vi "FPGA_I2C_AD7747_Write_Read.vi"(5 "SPI Command":string="0000", 6 "SelectDut":bool[][](array[boolean])=[[TRUE, TRUE, TRUE, TRUE, TRUE, TRUE, TRUE, TRUE, TRUE, TRUE, TRUE, TRUE, TRUE, TRUE, TRUE, TRUE, FALSE, FALSE, FALSE, FALSE, FALSE, FALSE, FALSE, FALSE, FALSE, FALSE, FALSE, FALSE, FALSE, FALSE, FALSE, FALSE], [TRUE, TRUE, TRUE, TRUE, TRUE, TRUE, TRUE, TRUE, TRUE, TRUE, TRUE, TRUE, TRUE, TRUE, TRUE, TRUE, FALSE, FALSE, FALSE, FALSE, FALSE, FALSE, FALSE, FALSE, FALSE, FALSE, FALSE, FALSE, FALSE, FALSE, FALSE, FALSE], [FALSE, FALSE, FALSE, FALSE, FALSE, FALSE, FALSE, FALSE, FALSE, FALSE, FALSE, FALSE, FALSE, FALSE, FALSE, FALSE, TRUE, FALSE, FALSE, FALSE, FALSE, FALSE, TRUE, FALSE, FALSE, FALSE, FALSE, FALSE, FALSE, FALSE, FALSE, TRUE], [FALSE, FALSE, FALSE, FALSE, FALSE, FALSE, FALSE, FALSE, FALSE, FALSE, FALSE, FALSE, FALSE, FALSE, FALSE, FALSE, TRUE, FALSE, FALSE, FALSE, FALSE, FALSE, TRUE, FALSE, FALSE, FALSE, FALSE, FALSE, FALSE, FALSE, FALSE, TRUE]], 7 "Stop":bool, 8 "error in":errorcluster, 9 "OFFSet Cal":bool, 10 "CapDac":bool, 11 "READ":bool) -> (0 "error out":errorcluster, 2 "Cap_Data":string[][](table)=[["0x02", "3.76992", "0x02", "3.77728"], ["0x02", "3.78382", "0x00", "-8.19200"], ["0x02", "3.94961", "0x02", "3.76741"], ["0x02", "4.54733", "0x02", "4.63408"], ["0x02", "3.84893", "0x02", "3.82712"], ["0x02", "3.80094", "0x02", "3.80246"], ["0x02", "3.79069", "0x02", "3.74972"], ["0x02", "3.80074", "0x02", "3.79936"], ["0x02", "4.04241", "0x02", "3.22665"], ["0x02", "3.79415", "0x02", "3.76417"], ["0x02", "3.79553", "0x02", "3.77940"], ["0x02", "1.03695", "0x02", "1.03735"], ["0x02", "3.80021", "0x02", "3.77078"], ["0x02", "4.65608", "0x02", "4.70829"], ["0x02", "3.74688", "0x02", "3.75749"], ["0x02", "3.81169", "0x02", "3.79781"]])   [LabVIEW 2012]
panel:
  out "Activity Log":string
  in  "Monitor":bool=TRUE
  in  "Write SPI":bool
  out "Simulate FPGA":bool
  out "Online":bool
  in  "SPI Clock Rate (Hz)":dbl=1000000.0 caption="Clock Rate" format="%.1p Hz"
  in  "I2C Slave Address":u8=144 caption="Slave Address" format="0x%02x"
  in  "I2C Clock Rate (Hz)":dbl=100000.0 caption="Clock Rate" format="%.0p Hz"
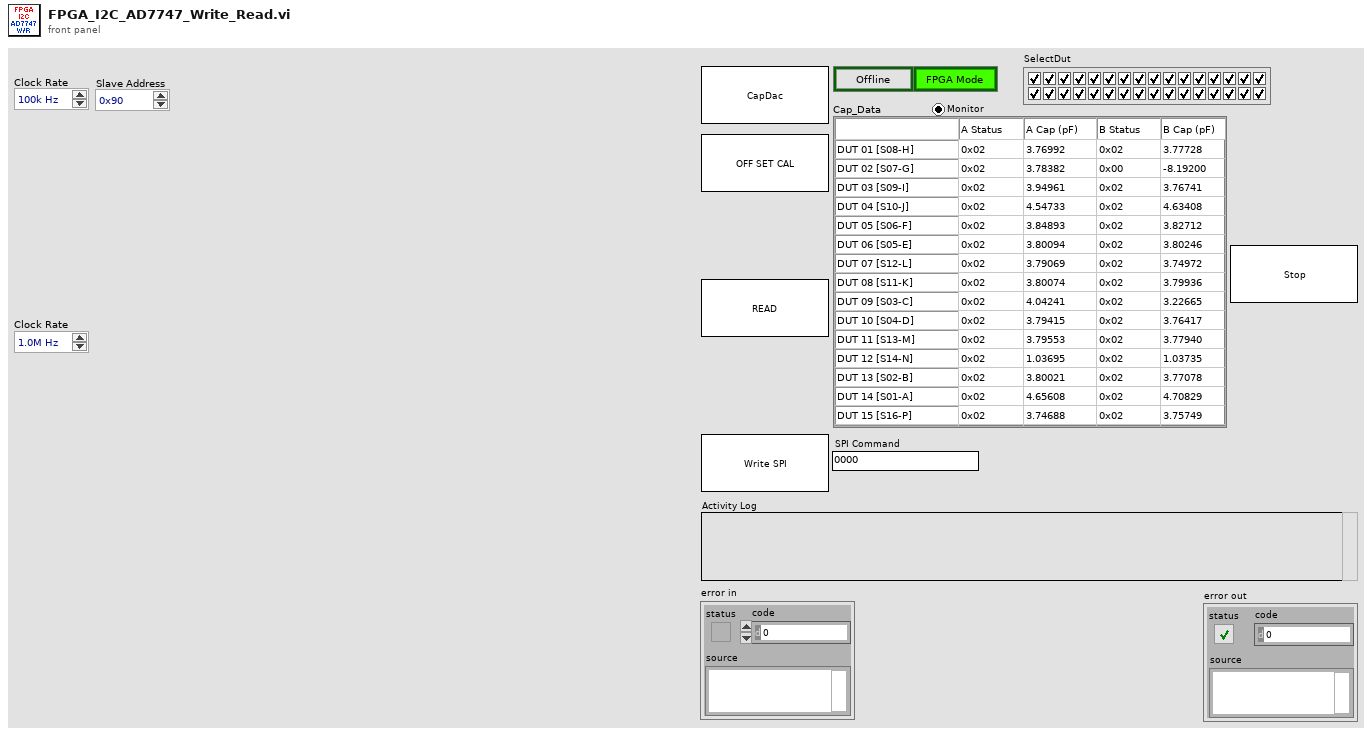
[diagram p1: front panel]
types:
  T1 = typedef "WSVCAP SHL Core System Cluster.ctl" = cluster{"Settings":T2, "FPGA Resource":tag, "Online":bool, "I2C Wait Ticks":u32, "SPI Wait Ticks":u32, "RFFE Wait Ticks":u32}
  T2 = typedef "WSVCAP SHL I2C Settings Cluster.ctl" = cluster{"FPGA Resource Name":string, "I2C Slave Address":u8, "I2C Clock Rate (Hz)":dbl, "SPI Clock Rate (Hz)":dbl, "RFFE Slave Address":u8, "RFFE Clock Rate (Hz)":dbl, "Simulate FPGA":bool}
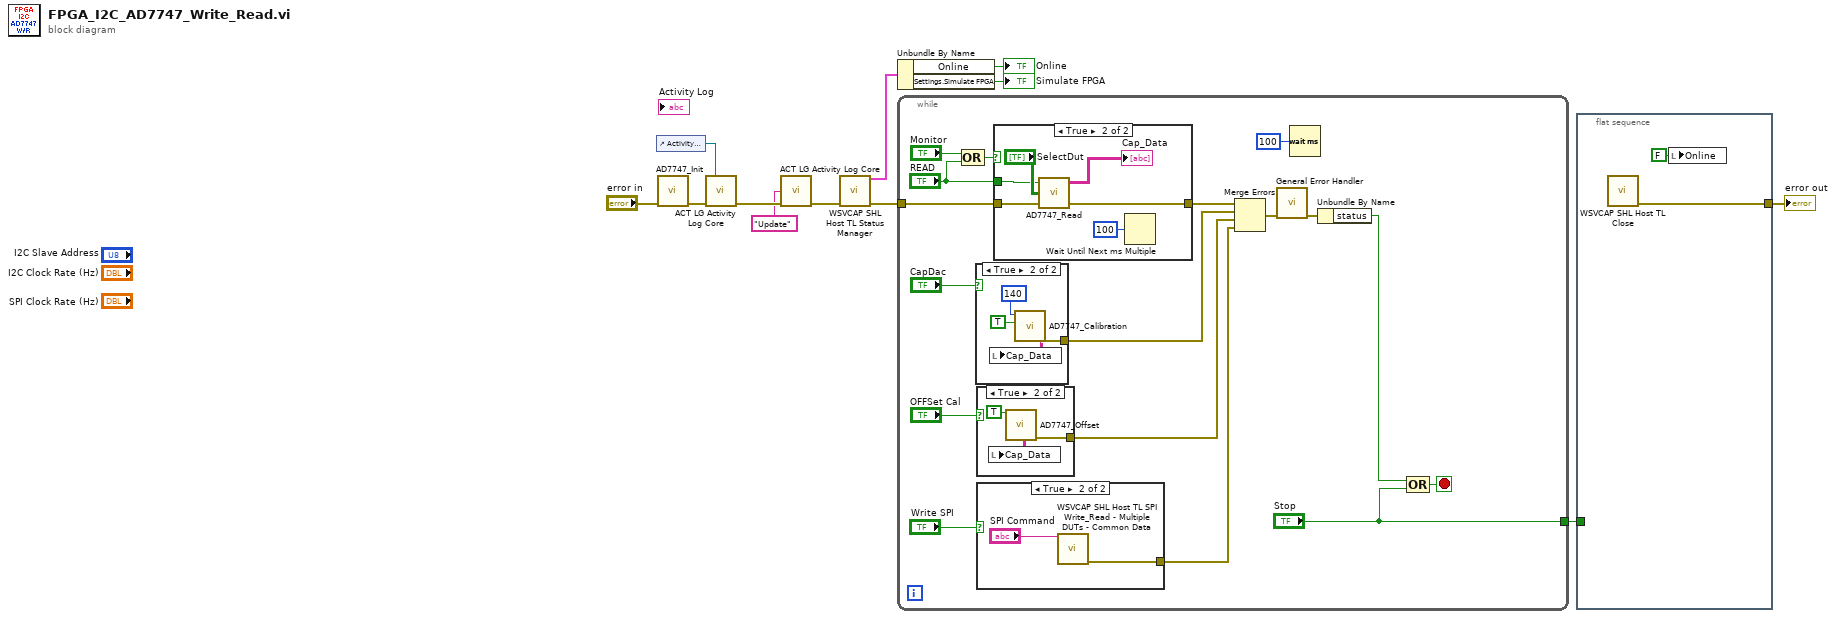
[diagram p0: block diagram]
diagram:
  n1 = control-ref of="Activity Log"() -> (w4:refnum<vi>)
  n2 = call "AD7747_Init.vi"("error in"="error in") -> ("error out"=w5:errorcluster)  [unwired: 10 in]
  n3 = call "ACT LG Activity Log Core.vi"("Display Ref"=w4, "Error In (no error)"=w5) -> ("Error Out"=w3:errorcluster)  [unwired: 12 in, 1 out]
  n4 = call "ACT LG Activity Log Core.vi"("Log Line"="Update", "Error In (no error)"=w3) -> ("Error Out"=w2:errorcluster)  [unwired: 12 in, 1 out]
  n5 = call "WSVCAP SHL Host TL Status Manager.vi"("error in"=w2) -> ("System Out"=w12:T1, "error out"=w7:errorcluster)  [unwired: 13 in]
  n6 = Unbundle By Name(w12) -> ("Online"=→"Online":bool, "Settings.Simulate FPGA"=→"Simulate FPGA":bool)
  n7 = while {
    tunnel: w7 -> [w23]
    tunnel: ["Stop"] -> w6
    stop <- w17 stop-if-true
    n8 = Compound Arithmetic op=OR("Monitor", "READ") -> (w14:bool)
    n9 = case shown="True" "CapDac" {
      tunnel: [_ w45] -> w28
      frame False {
      }
      frame True {
        n10 = call "AD7747_Calibration.vi"("Read After CapDac?"=TRUE, "Cap_Dac Value"=u8 140) -> ("errorout"=w45:errorcluster, "AD7747 Values"=w44:string[][])  [unwired: 8 in]
        n11 = local write "Cap_Data"(w44) -> ()
      }
    }
    n12 = case shown="True" "OFFSet Cal" {
      tunnel: [_ w41] -> w29
      frame False {
      }
      frame True {
        n13 = call "AD7747_Offset.vi"("Read?"=TRUE) -> ("error Out"=w41:errorcluster, "AD7747 Values"=w39:string[][])  [unwired: 9 in]
        n14 = local write "Cap_Data"(w39) -> ()
      }
    }
    n15 = case shown="True" "Write SPI" {
      tunnel: [_ w31] -> w24
      frame False {
      }
      frame True {
        n16 = call "WSVCAP SHL Host TL SPI Write_Read - Multiple DUTs - Common Data.vi"("Data Out"="SPI Command") -> ("error out"=w31:errorcluster)  [unwired: 13 in, 1 out]
      }
    }
    n17 = case shown="True" w14 {
      tunnel: w23 -> [w32 w38]
      tunnel: [w32 w37] -> w22
      tunnel: "READ" -> [_ w33]
      frame False {
      }
      frame True {
        n18 = call "AD7747_Read.vi"("error in"=w38, "DUT Mask Array (All)"="SelectDut", "Log (T)"=w33) -> ("error Out"=w37:errorcluster, "AD7747 Values"=→"Cap_Data":string[][])  [unwired: 1 in]
        n19 = Wait Until Next ms Multiple(millisecond multiple=u32 100) -> ()  [unwired: 1 out]
      }
    }
    n20 = Merge Errors(w22, w28, w29, w24) -> (w21:errorcluster)
    n21 = call <vilib>:"General Error Handler.vi"("error in (no error)"=w21) -> ("error out"=w19:errorcluster)  [unwired: 10 in, 4 out]
    n22 = Wait (ms)(milliseconds to wait=u32 100) -> ()  [unwired: 1 out]
    n23 = Unbundle By Name(w19) -> ("status"=w18:bool)
    n24 = Compound Arithmetic op=OR(w18, "Stop") -> (w17:bool)
  }
  n25 = flat-sequence {
    tunnel: [w46] -> w9
    tunnel: w6 -> [_]
    frame #0 {
      n26 = call "WSVCAP SHL Host TL Close.vi"() -> ("error out"=w46:errorcluster)  [unwired: 15 in]
      n27 = local write "Online"(FALSE ("Online")) -> ()
    }
  }
  "error out" <- w9
